vi "XML - Get Channel XML String.vi"(8 "error in (no error)":errorcluster, 11 "Channels":T1[](array[typedef]) {"Data Type" items=["U8", "U16", "U32", "U64", "I8", "I16", "I32", "I64", "SGL", "DBL", "EXT"]}) -> (0 "error out":errorcluster, 3 "Channels String":string)   [LabVIEW 2016, in "UDP-Custom-Device System Explorer.lvlib"]
uses:
  UDP-Custom-Device System Explorer.lvlib
  Types/XML/XML - Channel.ctl
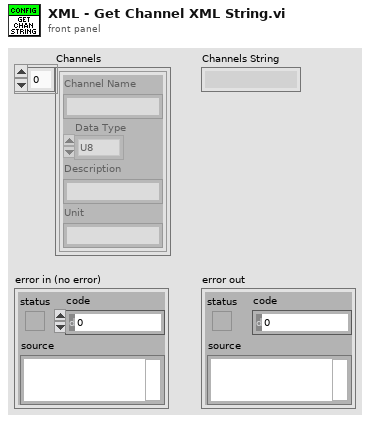
[diagram p1: front panel]
types:
  T1 = typedef "UDP-Custom-Device System Explorer.lvlib/XML - Channel.ctl" = cluster{"Channel Name":string, "Data Type":u16, "Description":string, "Unit":string}
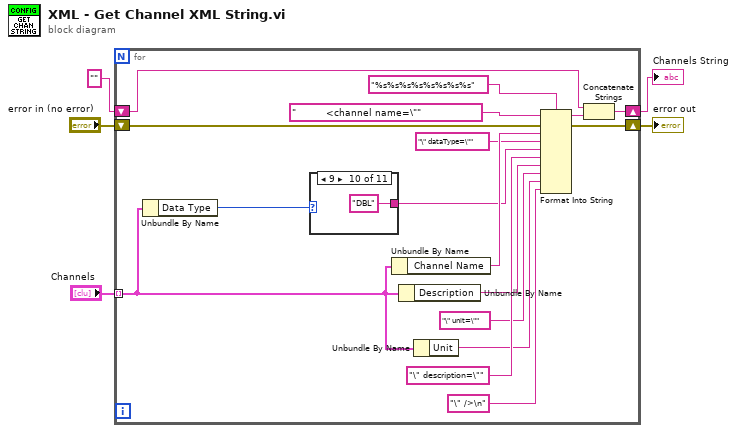
[diagram p0: block diagram]
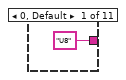
[diagram p2: hidden frame]
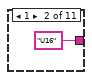
[diagram p3: hidden frame]
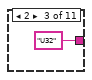
[diagram p4: hidden frame]
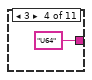
[diagram p5: hidden frame]
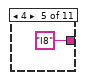
[diagram p6: hidden frame]
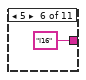
[diagram p7: hidden frame]
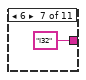
[diagram p8: hidden frame]
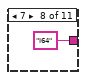
[diagram p9: hidden frame]
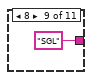
[diagram p10: hidden frame]
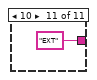
[diagram p11: hidden frame]
diagram:
  n1 = for {
    tunnel: "Channels" -> [w10] mode=indexing
    shift-right: [w6] -> w5
    shift-left: "error in (no error)" -> [w7]
    shift-right: [w9] -> w4
    shift-left: "" ("initial string") -> [w8]
    n2 = Unbundle By Name(w10) -> ("Data Type"=w18:u16)
    n3 = case shown="9" w18 {
      tunnel: ["U8" "U16" "U32" "U64" "I8" "I16" "I32" "I64" "SGL" "DBL" "EXT"] -> w17
      frame 0, Default {
      }
      frame 1 {
      }
      frame 2 {
      }
      frame 3 {
      }
      frame 4 {
      }
      frame 5 {
      }
      frame 6 {
      }
      frame 7 {
      }
      frame 8 {
      }
      frame 9 {
      }
      frame 10 {
      }
    }
    n4 = Unbundle By Name(w10) -> ("Channel Name"=w20:string)
    n5 = Unbundle By Name(w10) -> ("Description"=w15:string)
    n6 = Unbundle By Name(w10) -> ("Unit"=w13:string)
    n7 = Format Into String(format string="%s%s%s%s%s%s%s%s", initial string="          <channel name=\"", error in=w7, w20, "\" dataType=\"" ("input 2"), w17, "\" description=\"" ("input 2"), w15, "\" unit=\"" ("input 2"), w13, "\" />\n" ("input 2")) -> (resulting string=w22:string, error out=w6:errorcluster)
    n8 = Concatenate Strings(w8, w22) -> (w9:string)
  }
  "error out" <- w5
  "Channels String" <- w4
